vi "Select Mainframe 1.vi"(8 "error in (no error) 2":errorcluster, 11 "VISA resource name":refnum<visa-resource-name>) -> (0 "error out":errorcluster, 3 "VISA Refnum out":refnum<visa-resource-name>)   [LabVIEW 2018]
panel:
  out "Mainframe response":string
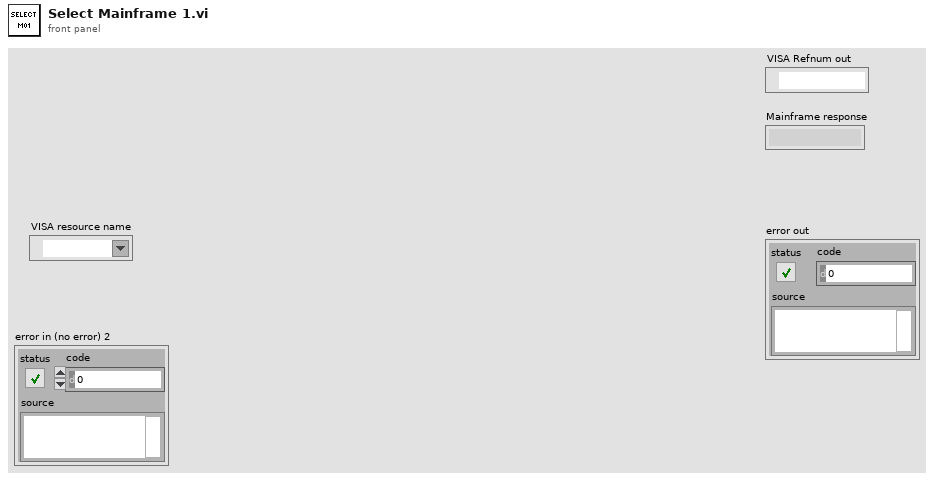
[diagram p1: front panel]
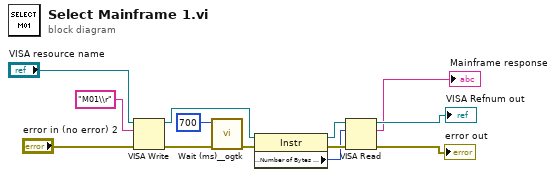
[diagram p0: block diagram]
diagram:
  n1 = VISA Write(VISA resource name="VISA resource name", write buffer="M01\\r" ("Mainframe"), error in (no error)="error in (no error) 2") -> (VISA resource name out=w6:refnum<visa-resource-name>, error out=w11:errorcluster)  [unwired: 1 out]
  n2 = call <userlib>:"Wait (ms)__ogtk.vi"("error in (no error)"=w11, "milliseconds to wait"=u32 700) -> ("error out"=w5:errorcluster)  [unwired: 8 in, 1 out]
  n3 = property class="Instr"(reference=w6, error in=w5) -> (reference out=w8:refnum<visa-resource-name>, error out=w9:errorcluster, "Serial Settings:Number of Bytes at Serial Port"=w7:u32)
  n4 = VISA Read(VISA resource name=w8, byte count=w7, error in (no error)=w9) -> (VISA resource name out=→"VISA Refnum out":refnum<visa-resource-name>, read buffer=→"Mainframe response":string, error out=→"error out":errorcluster)  [unwired: 1 out]
